vi "Populate PXI Trigger Bus Information.vi"(0 "hardware resources [channel]":T1[](array[typedef])=[{"7902R (Tx)"="TxFpga0", "3610 (Tx)"="Dac0", "3620 (IF)"="IF0", "3630 (RX)"="Adc0", "7902R (Rx)"="RxFpga0"}], 5 "hardware setup":T3, 11 "error in (no error)":errorcluster) -> (4 "hardware resources out":T1[](array[typedef])=[{"7902R (Tx)"="TxFpga0", "3610 (Tx)"="Dac0", "3620 (IF)"="IF0", "3630 (RX)"="Adc0", "7902R (Rx)"="RxFpga0"}], 6 "pxi trigger bus segment information [channel]":T5[](array[typedef]), 15 "error out":errorcluster)   [LabVIEW 2019]
uses:
  TypeDefs/Resources.ctl
  <vilib>/userdefined/High Color/nirio_resource_hc.ctl
  TypeDefs/PXI Trigger Bus Info.ctl
  TypeDefs/Hardware Configuration.ctl
  TypeDefs/Direction.ctl
  <vilib>/nisyscfg/Close (Filter).vi
  <vilib>/nisyscfg/Close (System).vi
  <vilib>/nisyscfg/nisyscfg.lvlib
  <resource>/objmgr/nicontrollersysapi.rc
  <resource>/objmgr/niflexrioatomicsae.rc
panel:
  in  "target (localhost)":refnum<k21>="localhost"
  out "devices info":T6(array[cluster])
  out "chassis/backplanes info":T7(array[cluster])
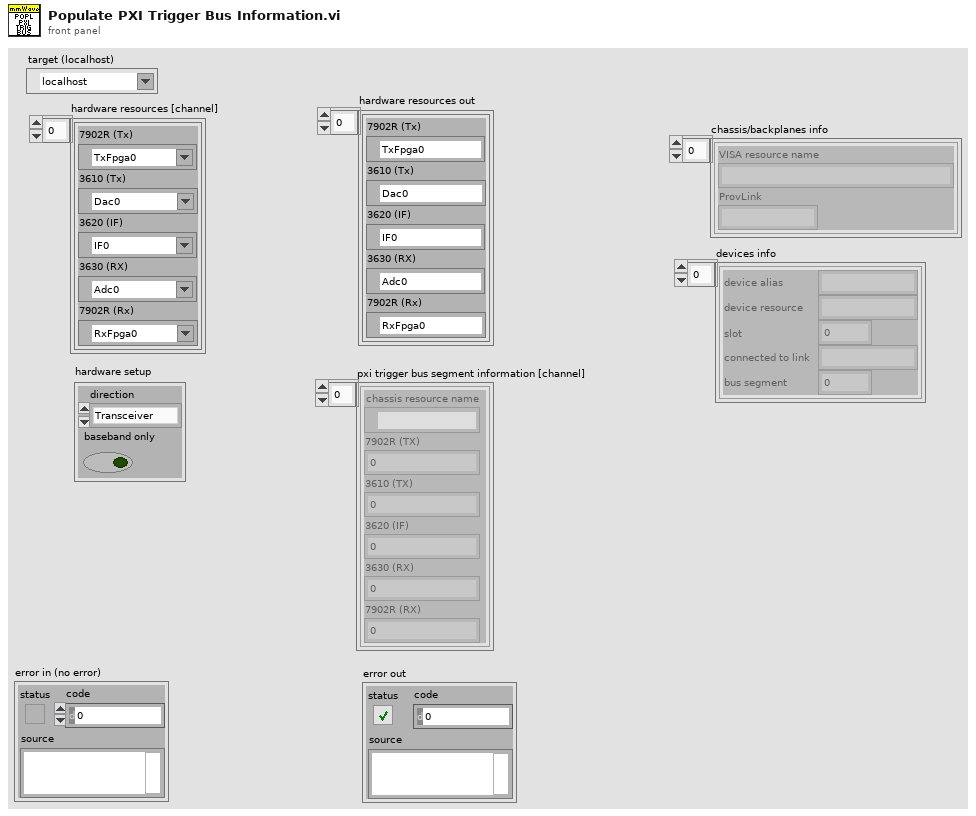
[diagram p1: front panel]
types:
  T1 = typedef "Resources.ctl" = cluster{"7902R (Tx)":T2, "3610 (Tx)":refnum<visa-resource-name>, "3620 (IF)":T2, "3630 (RX)":refnum<visa-resource-name>, "7902R (Rx)":T2}
  T2 = typedef "nirio_resource_hc.ctl" = tag
  T3 = typedef "Hardware Configuration.ctl" = cluster{"direction":T4, "baseband only":bool}
  T4 = typedef "Direction.ctl" = enum16{"Transceiver", "Receiver", "Transmitter"}
  T5 = typedef "PXI Trigger Bus Info.ctl" = cluster{"chassis resource name":refnum<visa-resource-name>, "7902R (TX)":i16, "3610 (TX)":i16, "3620 (IF)":i16, "3630 (RX)":i16, "7902R (RX)":i16}
  T6 = cluster{"device alias":string, "device resource":string, "slot":i32, "connected to link":string, "bus segment":i32}[]
  T7 = cluster{"VISA resource name":string, "ProvLink":string}[]
  T8 = cluster{"VISA resource name":string, "ProvLink":string}
  T9 = cluster{"device alias":string, "device resource":string, "slot":i32, "connected to link":string, "bus segment":i32}
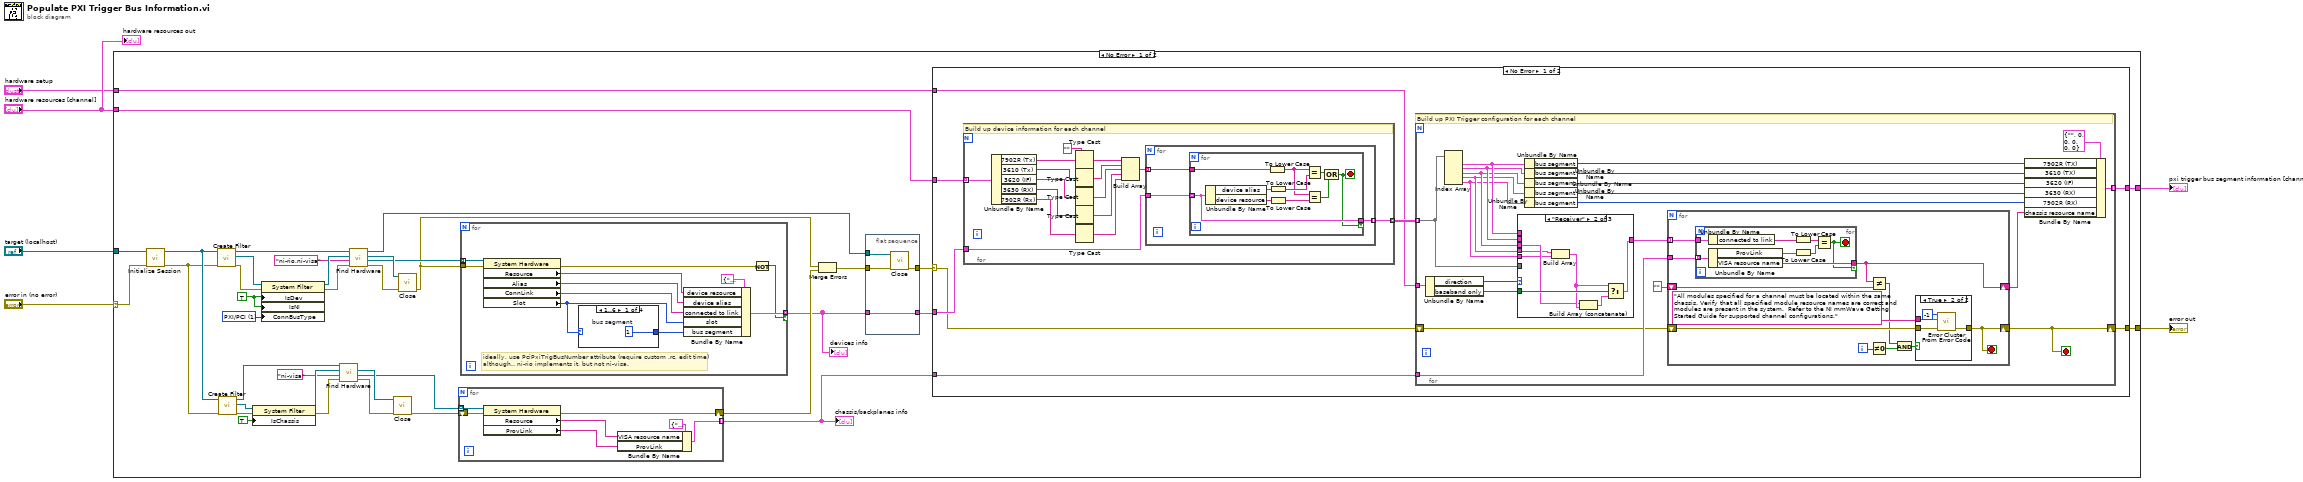
[diagram p0: block diagram]
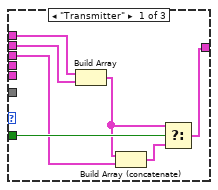
[diagram p2: hidden frame]
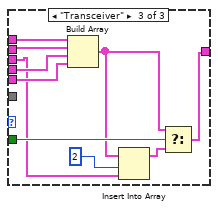
[diagram p3: hidden frame]
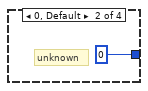
[diagram p6: hidden frame]
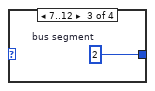
[diagram p7: hidden frame]
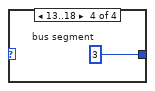
[diagram p8: hidden frame]
diagram:
  n1 = case shown="No Error" "error in (no error)" {
    selector: "error in (no error)" -> [w11 w178]
    tunnel: "target (localhost)" -> [w38 _]
    tunnel: "hardware resources [channel]" -> [w20 _]
    tunnel: [w15 _] -> w4
    tunnel: "hardware setup" -> [w13 _]
    tunnel: [w12 w178] -> w2
    frame No Error {
      w7 = u32 1 items=["BuiltIn/System", "PXI/PCI", "USB", "GPIB", "VXI", "Serial", "TCP/IP", "cRIO", "SCXI", "cDAQ", "SwitchBlock", "SCC", "FireWire", "Accessory", "CAN"] ("Devices & Chassis:Connects To Bus Type")
      w41 = TRUE ("Is Device")
      n2 = call <vilib>:"Initialize Session.vi"("error in (no error)"=w11, "Target (localhost)"=w38) -> ("error out"=w17:errorcluster, "Session out"=w32:refnum<k21>)  [unwired: 8 in]
      n3 = call <vilib>:"Create Filter.vi"("error in (no error)"=w17, "Session in"=w32) -> ("error out"=w44:errorcluster, "Filter out"=w43:refnum<k20>, "Session out"=w42:refnum<k21>)  [unwired: 7 in]
      n4 = call <vilib>:"Create Filter.vi"("error in (no error)"=w17, "Session in"=w32) -> ("error out"=w33:errorcluster, "Filter out"=w34:refnum<k20>, "Session out"=w30:refnum<k21>)  [unwired: 7 in]
      n5 = property class="System Filter"(reference=w34, error in=w33, "IsChassis"=TRUE ("Is Chassis")) -> (reference out=w29:refnum<k20>, error out=w28:errorcluster)
      n6 = property class="System Filter"(reference=w43, error in=w44, "IsDev"=w41, "IsNI"=w41, "ConnBusType"=w7) -> (reference out=w40:refnum<k20>, error out=w19:errorcluster)
      n7 = call <vilib>:"Find Hardware.vi"("error in (no error)"=w28, "Experts"="ni-visa", "Filter in"=w29, "Session in"=w30) -> ("error out"=w26:errorcluster, "Resources out"=w25:refnum<k20>[], "Filter out"=w27:refnum<k20>)  [unwired: 4 in, 1 out]
      n8 = call <vilib>:"Find Hardware.vi"("error in (no error)"=w19, "Experts"="ni-rio,ni-visa", "Filter in"=w40, "Session in"=w42) -> ("error out"=w18:errorcluster, "Resources out"=w36:refnum<k20>[], "Filter out"=w37:refnum<k20>, "Session out"=w35:refnum<k21>)  [unwired: 4 in]
      n9 = call-poly <vilib>:"Close.vi"("error in (no error)"=w26, "Filter in"=w27) -> ("error out"=w24:errorcluster)  [unwired: 9 in]
      n10 = call-poly <vilib>:"Close.vi"("error in (no error)"=w18, "Filter in"=w37) -> ("error out"=w10:errorcluster)  [unwired: 9 in]
      n11 = for {
        tunnel: w25 -> [w162] mode=indexing
        tunnel: [w158] -> w14 mode=indexing
        shift-right: [w157] -> w23
        shift-left: w24 -> [w161]
        n12 = property class="System Hardware"(reference=w162, error in=w161) -> (error out=w157:errorcluster, "Resource"=w160:string, "ProvLink"=w159:string)  [unwired: 1 out]
        n13 = Bundle By Name(cluster=T8 {"VISA resource name"="PXI0::1::BACKPLANE", "ProvLink"="PXI1"} ("chassis info"), "VISA resource name"=w160, "ProvLink"=w159) -> (w158:T8)
      }
      "chassis/backplanes info" <- w14
      n14 = for {
        tunnel: w36 -> [w171] mode=indexing
        tunnel: [w173] -> w8 mode=indexing if=w163
        tunnel: w10 -> [w170]
        # "ideally, use PciPxiTrigBusNumber attribute (require custom .rc, edit time)\nalthough.. ni-rio implements it, but not ni-visa."
        n15 = property class="System Hardware"(reference=w171, error in=w170) -> (error out=w164:errorcluster, "Resource"=w166:string, "Alias"=w167:string, "ConnLink"=w169:string, "Slot"=w168:i32)  [unwired: 1 out]
        n16 = case shown="1..6" w168 {
          tunnel: [w174 0 ("bus segment") w176 w177] -> w172
          frame 1..6 {
            w174 = 1  # bus segment
          }
          frame 0, Default {
            # "unknown"
          }
          frame 7..12 {
            w176 = 2  # bus segment
          }
          frame 13..18 {
            w177 = 3  # bus segment
          }
        }
        n17 = Bundle By Name(cluster=T9 {"device alias"="", "device resource"="", "slot"=0, "connected to link"="", "bus segment"=0} ("device info"), "device resource"=w166, "device alias"=w167, "connected to link"=w169, "slot"=w168, "bus segment"=w172) -> (w173:T9)
        n18 = Not(x=w164) -> (.not. x?=w163:bool)
      }
      "devices info" <- w8
      n19 = Merge Errors(w10, w23) -> (w22:errorcluster)
      n20 = flat-sequence {
        tunnel: w35 -> [w48]
        tunnel: w22 -> [w47]
        tunnel: [w46] -> w16
        tunnel: [w45] -> w9
        tunnel: w8 -> [w45]
        frame #0 {
          n21 = call-poly <vilib>:"Close.vi"("error in (no error)"=w47, "Session in"=w48) -> ("error out"=w46:errorcluster)  [unwired: 9 in]
        }
      }
      n22 = case shown="No Error" w16 {
        selector: w16 -> [w50 w155]
        tunnel: w20 -> [w56 _]
        tunnel: w9 -> [w55 _]
        tunnel: [w49 w155] -> w12
        tunnel: [w53 _] -> w15
        tunnel: w14 -> [w52 _]
        tunnel: w13 -> [w51 _]
        frame No Error {
          n23 = for {
            tunnel: w56 -> [w141] mode=indexing
            tunnel: w55 -> [w128]
            tunnel: [w127] -> w54 mode=indexing
            w139 = "" ("type")
            # "Build up device information for each channel"
            n24 = Unbundle By Name(w141) -> ("7902R (Tx)"=w140:T2, "3610 (Tx)"=w138:refnum<visa-resource-name>, "3620 (IF)"=w137:T2, "3630 (RX)"=w136:refnum<visa-resource-name>, "7902R (Rx)"=w135:T2)
            n25 = Type Cast(type=w139, x=w140) -> (*(type *) &x=w134:string)
            n26 = Type Cast(type=w139, x=w138) -> (*(type *) &x=w133:string)
            n27 = Type Cast(type=w139, x=w137) -> (*(type *) &x=w132:string)
            n28 = Type Cast(type=w139, x=w136) -> (*(type *) &x=w131:string)
            n29 = Type Cast(type=w139, x=w135) -> (*(type *) &x=w130:string)
            n30 = Build Array(w134, w133, w132, w131, w130) -> (w129:string[])
            n31 = for {
              tunnel: w129 -> [w143] mode=indexing
              tunnel: w128 -> [w144]
              tunnel: [w142] -> w127 mode=indexing
              n32 = for {
                tunnel: w144 -> [w154] mode=indexing
                tunnel: w143 -> [w153]
                tunnel: [w154] -> w142 if=w145
                stop <- w145 stop-if-true
                n33 = Unbundle By Name(w154) -> ("device alias"=w152:string, "device resource"=w150:string)
                n34 = To Lower Case(string=w153) -> (all lower case string=w148:string)
                n35 = To Lower Case(string=w152) -> (all lower case string=w151:string)
                n36 = To Lower Case(string=w150) -> (all lower case string=w149:string)
                n37 = Equal?(x=w148, y=w151) -> (x = y?=w146:bool)
                n38 = Equal?(x=w148, y=w149) -> (x = y?=w147:bool)
                n39 = Compound Arithmetic op=OR(w146, w147) -> (w145:bool)
              }
            }
          }
          n40 = for {
            tunnel: w54 -> [w71] mode=indexing
            tunnel: [w73] -> w53 mode=indexing
            tunnel: w52 -> [w62]
            tunnel: w51 -> [w72]
            shift-right: [w58] -> w49
            shift-left: w50 -> [w60]
            stop <- w58 stop-if-true
            # "Build up PXI Trigger configuration for each channel"
            n41 = Unbundle By Name(w72) -> ("direction"=w70:T4, "baseband only"=w69:bool)
            n42 = Index Array(array=w71) -> (element #1=w68:T9, element #2=w67:T9, element #3=w66:T9, element #4=w65:T9, element #5=w64:T9)  [unwired: 5 in]
            n43 = case shown="\"Receiver\"" w70 {
              tunnel: w71 -> [_ _ _]
              tunnel: w69 -> [w83 w92 w102]
              tunnel: w68 -> [w85 _ w98]
              tunnel: w67 -> [w84 _ w97]
              tunnel: w66 -> [w81 w90 w94]
              tunnel: w65 -> [_ w87 w100]
              tunnel: w64 -> [_ w86 w99]
              tunnel: [w79 w88 w101] -> w63
              frame "Transmitter" {
                n44 = Build Array(w85, w84) -> (w82:T6)
                n45 = Build Array (concatenate)(w82, w81) -> (w80:T6)
                n46 = Select(t=w82, s=w83, f=w80) -> (s? t:f=w79:T6)
              }
              frame "Receiver" {
                n47 = Build Array(w87, w86) -> (w91:T6)
                n48 = Build Array (concatenate)(w90, w91) -> (w89:T6)
                n49 = Select(t=w91, s=w92, f=w89) -> (s? t:f=w88:T6)
              }
              frame "Transceiver" {
                n50 = Build Array(w98, w97, w100, w99) -> (w96:T6)
                n51 = Insert Into Array(array=w96, index=2, new element=w94) -> (w93:T6)
                n52 = Select(t=w96, s=w102, f=w93) -> (s? t:f=w101:T6)
              }
            }
            n53 = Unbundle By Name(w68) -> ("bus segment"=w78:i32)
            n54 = Unbundle By Name(w67) -> ("bus segment"=w77:i32)
            n55 = Unbundle By Name(w66) -> ("bus segment"=w76:i32)
            n56 = Unbundle By Name(w65) -> ("bus segment"=w75:i32)
            n57 = Unbundle By Name(w64) -> ("bus segment"=w74:i32)
            n58 = for {
              tunnel: w63 -> [w103] mode=indexing
              tunnel: w62 -> [w113]
              shift-right: [w104] -> w59
              shift-left: "" ("VISA resource name") -> [w112]
              shift-right: [w105] -> w58
              shift-left: w60 -> [w110]
              i -> [w109]
              stop <- w105 stop-if-true
              n59 = for {
                tunnel: w103 -> [w123]
                tunnel: w113 -> [w126] mode=indexing
                tunnel: [w125] -> w104 if=w124
                stop <- w124 stop-if-true
                n60 = Unbundle By Name(w123) -> ("connected to link"=w122:string)
                n61 = Unbundle By Name(w126) -> ("ProvLink"=w119:string, "VISA resource name"=w125:string)
                n62 = To Lower Case(string=w122) -> (all lower case string=w121:string)
                n63 = To Lower Case(string=w119) -> (all lower case string=w120:string)
                n64 = Equal?(x=w121, y=w120) -> (x = y?=w124:bool)
              }
              n65 = Not Equal?(x=w104, y=w112) -> (x != y?=w107:bool)
              n66 = Not Equal To 0?(x=w109) -> (x != 0?=w108:bool)
              n67 = Compound Arithmetic op=AND(w107, w108) -> (w106:bool)
              n68 = case shown="True" w106 {
                tunnel: "All modules specified for a channel must be located within the same chassis. Verify that all specified module resource names are correct and modules are present in the system.  Refer to the NI mmWave Getting Started Guide for supported channel configurations." ("error message (\"\")") -> [_ w117]
                tunnel: w110 -> [w114 w116]
                tunnel: [w114 w115] -> w105
                frame False {
                }
                frame True {
                  n69 = call <vilib>:"Error Cluster From Error Code.vi"("error in (no error)"=w116, "error message (\"\")"=w117, "error code (0)"=-1) -> ("error out"=w115:errorcluster)  [unwired: 6 in]
                }
              }
            }
            n70 = Bundle By Name(cluster=T5 {"chassis resource name"="", "7902R (TX)"=0, "3610 (TX)"=0, "3620 (IF)"=0, "3630 (RX)"=0, "7902R (RX)"=0} ("pxi trigger bus information"), "7902R (TX)"=w78, "3610 (TX)"=w77, "3620 (IF)"=w76, "3630 (RX)"=w75, "7902R (RX)"=w74, "chassis resource name"=w59) -> (w73:T5)
          }
        }
        frame Error {
        }
      }
    }
    frame Error {
    }
  }
  "pxi trigger bus segment information [channel]" <- w4
  "error out" <- w2
  "hardware resources out" <- "hardware resources [channel]"
